vi "GetFrontPanelImage.vi"(7 "LabVIEW Web Service Request":refnum<class "Web Request.lvclass">) -> ()   [LabVIEW 2016]
uses:
  <vilib>/wsapi/Web Request.lvclass
  <vilib>/wsapi/NI_WebServices.lvlib
panel:
  # "Use the Web Service Request input terminal to call the VIs on the Web Services palette. Do not remove it from the connector pane unless you don't need access to the palette."
  # "Each additional control wired to the connector pane will be available as an input in the URL. To include an indicator in terminal-mode output (the default setting), it must also be wired to the connector pane."
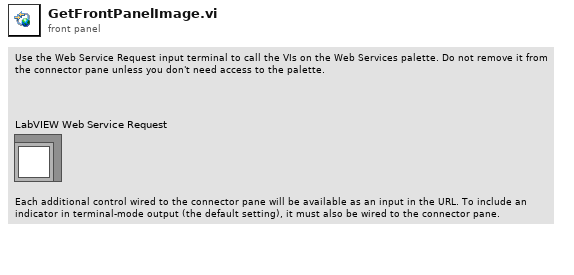
[diagram p1: front panel]
types:
  T1 = typedef "imagedata.ctl" = cluster{"image type":i32, "image depth":i32, "image":u8[], "mask":u8[], "colors":u32[], "Rectangle":cluster{"left":i16, "top":i16, "right":i16, "bottom":i16}}
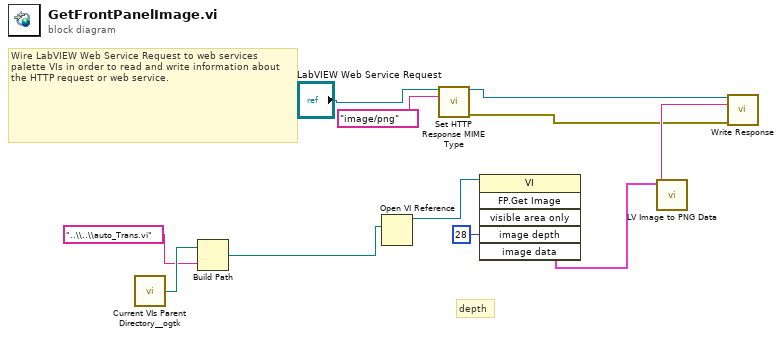
[diagram p0: block diagram]
diagram:
  # "depth"
  # "Wire LabVIEW Web Service Request to web services palette VIs in order to read and write information about the HTTP request or web service."
  n1 = call <userlib>:"Current VIs Parent Directory__ogtk.vi"() -> ("Parent Directory (+ Relative)"=w4:path)  [unwired: 5 in]
  n2 = Build Path(base path=w4, name or relative path="..\\..\\auto_Trans.vi") -> (appended path=w2:path)
  n3 = Open VI Reference(vi path=w2) -> (vi reference=w7:refnum<vi>)  [unwired: 5 in, 1 out]
  n4 = call <vilib>:"Set HTTP Response MIME Type.vi"("LabVIEW Web Service Request"="LabVIEW Web Service Request", "MIME type (text/html)"="image/png") -> ("LabVIEW Web Service Request out"=w10:refnum<class "Web Request.lvclass">, "error out"=w8:errorcluster)  [unwired: 12 in]
  n5 = invoke class="VI" method="FP.Get Image"(reference=w7, "image depth"=28 ("Image Depth")) -> ("image data"=w6:T1)  [unwired: 4 in, 5 out]
  n6 = call <vilib>:"LV Image to PNG Data.vi"("image data"=w6) -> ("png data"=w9:string)  [unwired: 9 in, 1 out]
  n7 = call <vilib>:"Write Response.vi"("LabVIEW Web Service Request"=w10, "response string"=w9, "error in (no error)"=w8) -> ()  [unwired: 11 in, 2 out]
